vi "GetSQLstring1.vi"(8 "错误输入":errorcluster, 11 "联机模式":enum16{"单机", "追溯"}(ring)) -> (0 "错误输出":errorcluster, 3 "连接字符串":string)   [LabVIEW 2020]
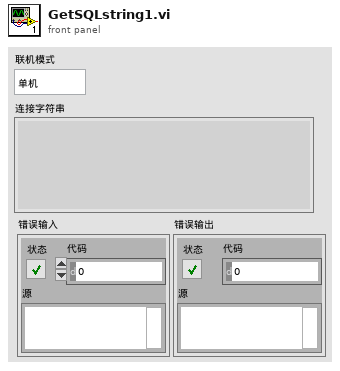
[diagram p1: front panel]
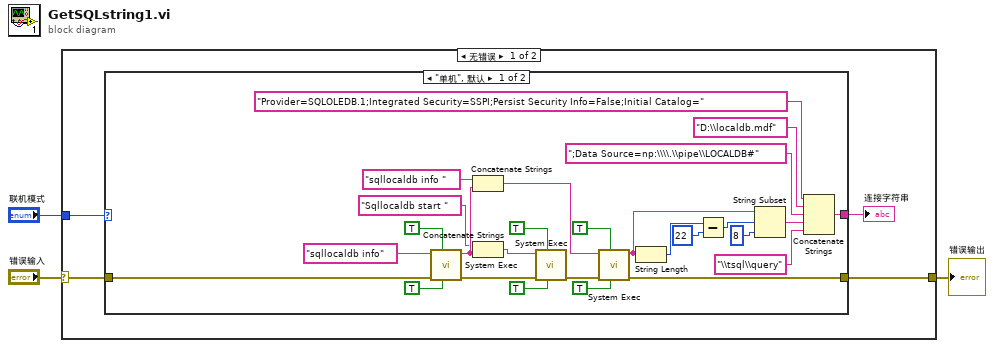
[diagram p0: block diagram]
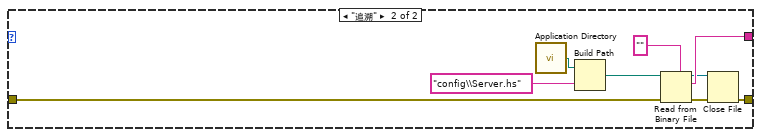
[diagram p2: hidden frame]
diagram:
  n1 = case shown="无错误" "错误输入" {
    selector: "错误输入" -> [w5 w44]
    tunnel: [w6 w44] -> w3
    tunnel: "联机模式" -> [w4 _]
    frame No Error {
      n2 = case shown="\"单机\", 默认" w4 {
        tunnel: [w8 w39] -> w7
        tunnel: [w9 w36] -> w6
        tunnel: w5 -> [w10 w35]
        frame "单机", Default {
          n3 = call <vilib>:"System Exec.vi"("run minimized? (F)"=TRUE, "wait until completion? (T)"=TRUE, "error in (no error)"=w10, "command line"="sqllocaldb info") -> ("error out"=w33:errorcluster, "standard output"=w32:string)  [unwired: 4 in, 2 out]
          n4 = Concatenate Strings("sqllocaldb info " ("command line"), w32) -> (w30:string)
          n5 = Concatenate Strings("Sqllocaldb start " ("command line"), w32) -> (w31:string)
          n6 = call <vilib>:"System Exec.vi"("run minimized? (F)"=TRUE, "wait until completion? (T)"=TRUE, "error in (no error)"=w33, "command line"=w31) -> ("error out"=w34:errorcluster)  [unwired: 4 in, 3 out]
          n7 = call <vilib>:"System Exec.vi"("run minimized? (F)"=TRUE, "wait until completion? (T)"=TRUE, "error in (no error)"=w34, "command line"=w30) -> ("error out"=w9:errorcluster, "standard output"=w26:string)  [unwired: 4 in, 2 out]
          n8 = String Length(string=w26) -> (length=w27:i32)
          n9 = Subtract(x=w27, y=22) -> (x-y=w28:i32)
          n10 = String Subset(string=w26, offset (0)=w28, length (rest)=8 ("长度（剩余）")) -> (substring=w29:string)
          n11 = Concatenate Strings("Provider=SQLOLEDB.1;Integrated Security=SSPI;Persist Security Info=False;Initial Catalog=", "D:\\localdb.mdf", ";Data Source=np:\\\\.\\pipe\\LOCALDB#", w29, "\\tsql\\query") -> (w8:string)
        }
        frame "追溯" {
          n12 = call <vilib>:"Application Directory.vi"() -> ("Application Directory"=w43:path)
          n13 = Build Path(base path=w43, name or relative path="config\\Server.hs" ("名称或相对路径")) -> (appended path=w41:path)
          n14 = Read from Binary File(5:"", 8:w35, 11:w41) -> (0:w37:errorcluster, 2:w39:string, 3:w38:refnum<file>)  [unwired: 3 in, 1 out]
          n15 = Close File(refnum=w38, error in=w37) -> (error out=w36:errorcluster)  [unwired: 1 out]
        }
      }
      "连接字符串" <- w7
    }
    frame Error {
    }
  }
  "错误输出" <- w3
